vi "Set MAX soft position.vi"(0 "Zaber":T1={"Serial port handle"="", "Axis"="", "Controller #"=0, "Min position"=0.0, "Max position"=0.0, "Min velocity"=0.0, "Max velocity"=0.0, "Firmware"="", "Device ID"=0, "Variable event"=refnum, "Variable ref"=refnum, "Resolution, usteps/step"=0, "Serial port semaphore"=refnum, "Joystick buttons"={"MinDir"=1, "MaxDir"=2, "MedSpeed"=5, "HighSpeed"=6}} {"Joystick buttons"."HighSpeed" min=1 max=25 step=1; "Joystick buttons"."MedSpeed" min=1 max=25 step=1; "Joystick buttons"."MaxDir" min=1 max=25 step=1; "Joystick buttons"."MinDir" min=1 max=25 step=1}, 2 "Max soft position":dbl, 5 "error in":errorcluster) -> (14 "Zaber out":T1={"Serial port handle"="", "Axis"="", "Controller #"=0, "Min position"=0.0, "Max position"=0.0, "Min velocity"=0.0, "Max velocity"=0.0, "Firmware"="", "Device ID"=0, "Variable event"=refnum, "Variable ref"=refnum, "Resolution, usteps/step"=0, "Serial port semaphore"=refnum, "Joystick buttons"={"MinDir"=1, "MaxDir"=2, "MedSpeed"=5, "HighSpeed"=6}} {"Joystick buttons"."HighSpeed" min=1 max=25 step=1; "Joystick buttons"."MedSpeed" min=1 max=25 step=1; "Joystick buttons"."MaxDir" min=1 max=25 step=1; "Joystick buttons"."MinDir" min=1 max=25 step=1}, 16 "Max soft position":dbl, 19 "error out":errorcluster)   [LabVIEW 2018]
uses:
  Zaber.ctl
  GenericDataEvent/GenericEvent.ctl
  ZaberVariables.ctl
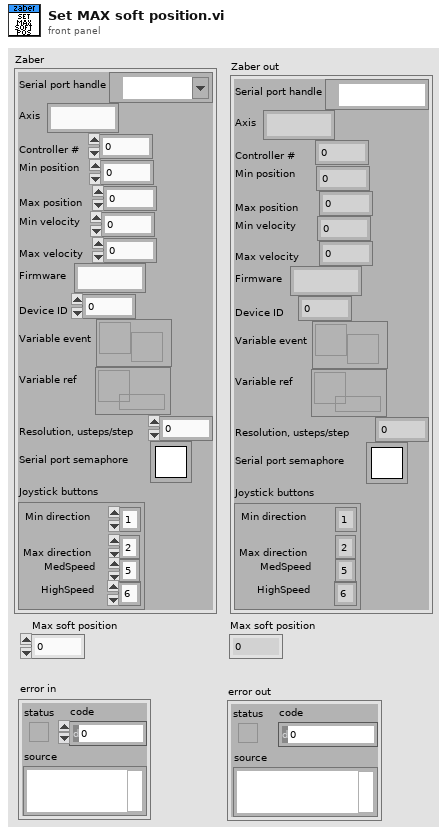
[diagram p1: front panel]
types:
  T1 = typedef "Zaber.ctl" = cluster{"Serial port handle":refnum<visa-resource-name>, "Axis":string, "Controller #":u8, "Min position":dbl, "Max position":dbl, "Min velocity":dbl, "Max velocity":dbl, "Firmware":string, "Device ID":i32, "Variable event":T2, "Variable ref":refnum<data-value>, "Resolution, usteps/step":i32, "Serial port semaphore":T3, "Joystick buttons":cluster{"MinDir":i32, "MaxDir":i32, "MedSpeed":i32, "HighSpeed":i32}}
  T2 = typedef "GenericEvent.ctl" = refnum<user-event>
  T3 = typedef "Semaphore RefNum" = refnum<k1>
  T4 = typedef "ZaberVariables.ctl" = cluster{"Position":i32, "Speed":i32, "Min soft position":dbl, "Max soft position":dbl, "Accelaration":i32}
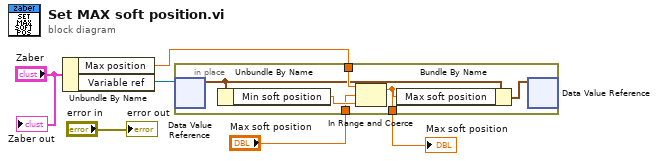
[diagram p0: block diagram]
diagram:
  n1 = Unbundle By Name("Zaber") -> ("Max position"=w3:dbl, "Variable ref"=w4:refnum<data-value>)
  n2 = in-place {
    in-place-border: w3 -> [w12]
    in-place-border: "Max soft position" -> [w10]
    in-place-border: [w7] -> w1
    n3 = in-place-dvr #1(w4) -> (w9:T4)  [unwired: 1 out]
    n4 = Unbundle By Name(w9) -> ("Min soft position"=w11:dbl)
    n5 = In Range and Coerce(upper limit=w12, x=w10, lower limit=w11) -> (coerced(x)=w7:dbl)  [unwired: 1 out]
    n6 = Bundle By Name(cluster=w9, "Max soft position"=w7) -> (w8:T4)
    n7 = in-place-dvr #1(w8) -> ()  [unwired: 2 out]
  }
  "Max soft position" <- w1
  "error out" <- "error in"
  "Zaber out" <- "Zaber"
